vi "Stanford Research 844 Buffer Measurement.vi"(0 "VISA Resource Name":refnum<visa-resource-name>, 2 "Data Sample Rate (10: 64 Hz)":u16(ring)=10 items=["62.5 mHz", "125 mHz", "250 mHz", "500 mHz", "1 Hz", "2 Hz", "4 Hz", "8 Hz", "16 Hz", "32 Hz", "64 Hz", "128 Hz", "256 Hz", "512 Hz", "Trigger"], 3 "Number Of Points (10)":i16=10, 8 "Channel 1 Display (0: X)":u16(ring) items=["X", "R [Volts rms]", "R [dBm]", "X noise", "AUX IN 1"], 10 "Channel 2 Display (0: Y)":u16(ring) items=["Y", "Phi", "Y noise [Volts]", "Y noise [dBm]", "AUX IN 2"]) -> (15 "Display CH1 Value":dbl format="%.2e", 16 "Display CH2 Value":dbl format="%.2e", 17 "Channel 1 Output Array":dbl[](array[numeric]) format="%.5f", 18 "Channel 2 Output Array":dbl[](array[numeric]) format="%.5f")   [LabVIEW 2010]
doc: "This VI shows how to acquire data and then transfer them in the buffered mode."
uses:
  <instrlib>/Stanford Research 844/Stanford Research 844.lvlib
panel:
  # "© 2005 National Instruments.  ALL RIGHTS RESERVED."
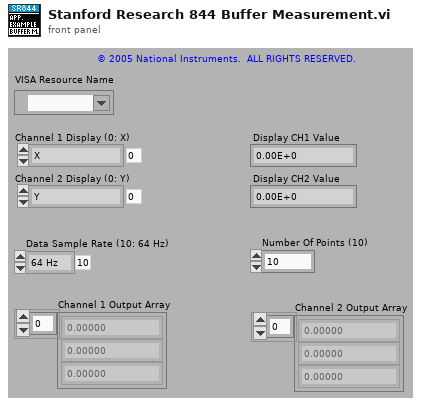
[diagram p1: front panel]
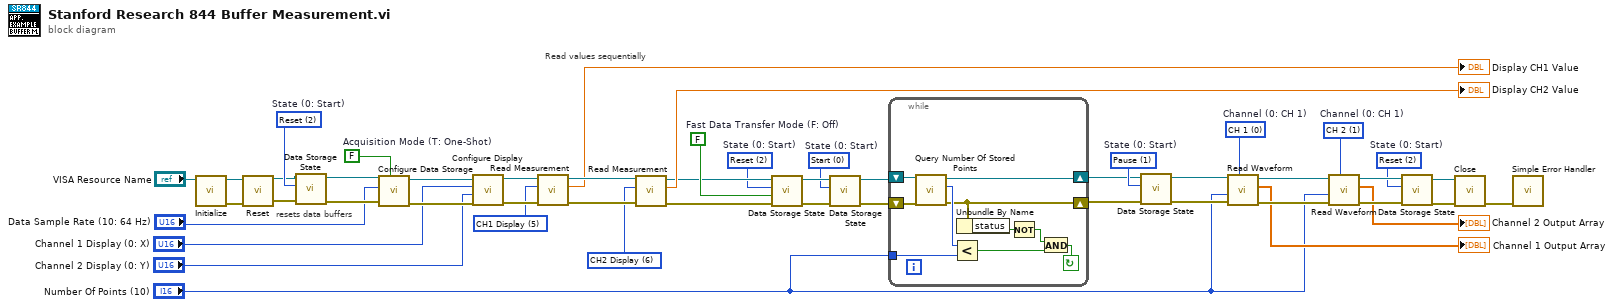
[diagram p0: block diagram]
diagram:
  w13 = FALSE  # Acquisition Mode (T: One-Shot)
  w19 = u16 6 items=["X", "Y", "R [V]", "R [dBm]", "Phi", "CH1 Display", "CH2 Display", "AUX 1", "AUX 2"] ("Value Selection (0: X)")
  w20 = u16 5 items=["X", "Y", "R [V]", "R [dBm]", "Phi", "CH1 Display", "CH2 Display", "AUX 1", "AUX 2"] ("Value Selection (0: X)")
  w23 = u16 2 items=["Start", "Pause", "Reset"]  # State (0: Start)
  w15 = u16 1 items=["CH 1", "CH 2"]  # Channel (0: CH 1)
  w16 = u16 0 items=["CH 1", "CH 2"]  # Channel (0: CH 1)
  w30 = u16 1 items=["Start", "Pause", "Reset"]  # State (0: Start)
  w32 = u16 0 items=["Start", "Pause", "Reset"]  # State (0: Start)
  w35 = u16 2 items=["Start", "Pause", "Reset"]  # State (0: Start)
  w44 = FALSE  # Fast Data Transfer Mode (F: Off)
  w49 = u16 2 items=["Start", "Pause", "Reset"]  # State (0: Start)
  # "resets data buffers"
  # "Read values sequentially"
  n1 = call <instrlib>:"Initialize.vi"("VISA Resource Name"="VISA Resource Name") -> ("error out"=w2:errorcluster, "VISA Resource Name Out"=w3:refnum<visa-resource-name>)  [unwired: 9 in]
  n2 = call <instrlib>:"Reset.vi"("VISA Resource Name"=w3, "error in (no error)"=w2) -> ("VISA Resource Name Out"=w12:refnum<visa-resource-name>, "error out"=w11:errorcluster)  [unwired: 12 in]
  n3 = call <instrlib>:"Data Storage State.vi"("Error In (no error)"=w11, "State (0: Start)"=w49, "VISA Resource Name"=w12) -> ("Error Out"=w47:errorcluster, "VISA Resource Name Out"=w48:refnum<visa-resource-name>)  [unwired: 7 in]
  n4 = call <instrlib>:"Configure Data Storage.vi"("Acquisition Mode (T: One-Shot)"=w13, "Error In (no error)"=w47, "Data Sample Rate (0: 62.5 mHz)"="Data Sample Rate (10: 64 Hz)", "VISA Resource Name"=w48) -> ("Error Out"=w45:errorcluster, "VISA Resource Name Out"=w46:refnum<visa-resource-name>)  [unwired: 6 in]
  n5 = call <instrlib>:"Configure Display.vi"("Error In (no error)"=w45, "Channel 2 Display (0: Y)"="Channel 2 Display (0: Y)", "Channel 1 Display (0: X)"="Channel 1 Display (0: X)", "VISA Resource Name"=w46) -> ("Error Out"=w42:errorcluster, "VISA Resource Name Out"=w43:refnum<visa-resource-name>)  [unwired: 6 in]
  n6 = call <instrlib>:"Read Measurement.vi"("Error In (no error)"=w42, "Value Selection (0: X)"=w20, "VISA Resource Name"=w43) -> ("Error Out"=w40:errorcluster, "Value"=→"Display CH1 Value":dbl, "VISA Resource Name Out"=w41:refnum<visa-resource-name>)  [unwired: 6 in]
  n7 = call <instrlib>:"Read Measurement.vi"("Error In (no error)"=w40, "Value Selection (0: X)"=w19, "VISA Resource Name"=w41) -> ("Error Out"=w36:errorcluster, "Value"=→"Display CH2 Value":dbl, "VISA Resource Name Out"=w37:refnum<visa-resource-name>)  [unwired: 6 in]
  n8 = call <instrlib>:"Data Storage State.vi"("Error In (no error)"=w36, "Fast Data Transfer Mode (F: Off)"=w44, "State (0: Start)"=w35, "VISA Resource Name"=w37) -> ("Error Out"=w33:errorcluster, "VISA Resource Name Out"=w34:refnum<visa-resource-name>)  [unwired: 6 in]
  n9 = call <instrlib>:"Data Storage State.vi"("Error In (no error)"=w33, "State (0: Start)"=w32, "VISA Resource Name"=w34) -> ("Error Out"=w9:errorcluster, "VISA Resource Name Out"=w10:refnum<visa-resource-name>)  [unwired: 7 in]
  n10 = while {
    tunnel: "Number Of Points (10)" -> [w57]
    shift-right: [w59] -> w8
    shift-left: w10 -> [w56]
    shift-right: [w54] -> w7
    shift-left: w9 -> [w55]
    stop <- w50 continue-if-true
    n11 = call <instrlib>:"Query Number Of Stored Points.vi"("Error In (no error)"=w55, "VISA Resource Name"=w56) -> ("Error Out"=w54:errorcluster, "Number Of Points"=w58:i16, "VISA Resource Name Out"=w59:refnum<visa-resource-name>)  [unwired: 7 in]
    n12 = Less?(x=w58, y=w57) -> (x < y?=w51:bool)
    n13 = Unbundle By Name(w54) -> ("status"=w52:bool)
    n14 = Not(x=w52) -> (.not. x?=w53:bool)
    n15 = And(x=w53, y=w51) -> (x .and. y?=w50:bool)
  }
  n16 = call <instrlib>:"Data Storage State.vi"("Error In (no error)"=w7, "State (0: Start)"=w30, "VISA Resource Name"=w8) -> ("Error Out"=w28:errorcluster, "VISA Resource Name Out"=w29:refnum<visa-resource-name>)  [unwired: 7 in]
  n17 = call <instrlib>:"Read Waveform.vi"("Channel (0: CH 1)"=w16, "Error In (no error)"=w28, "Number Of Points (1)"="Number Of Points (10)", "VISA Resource Name"=w29) -> ("Error Out"=w26:errorcluster, "Output Array"=→"Channel 1 Output Array":dbl[], "VISA Resource Name Out"=w27:refnum<visa-resource-name>)  [unwired: 5 in]
  n18 = call <instrlib>:"Read Waveform.vi"("Channel (0: CH 1)"=w15, "Error In (no error)"=w26, "Number Of Points (1)"="Number Of Points (10)", "VISA Resource Name"=w27) -> ("Error Out"=w24:errorcluster, "Output Array"=→"Channel 2 Output Array":dbl[], "VISA Resource Name Out"=w25:refnum<visa-resource-name>)  [unwired: 5 in]
  n19 = call <instrlib>:"Data Storage State.vi"("Error In (no error)"=w24, "State (0: Start)"=w23, "VISA Resource Name"=w25) -> ("Error Out"=w5:errorcluster, "VISA Resource Name Out"=w6:refnum<visa-resource-name>)  [unwired: 7 in]
  n20 = call <instrlib>:"Close.vi"("error in (no error)"=w5, "VISA Resource Name"=w6) -> ("error out"=w4:errorcluster)  [unwired: 9 in]
  n21 = call <vilib>:"Simple Error Handler.vi"("error in (no error)"=w4) -> ()  [unwired: 4 in, 5 out]
